vi "CloseCamera.vi"(8 "error in (no error)":errorcluster, 11 "HamaCam in":refnum<class "HamaCam.lvclass">) -> (0 "error out":errorcluster, 3 "HamaCam out":refnum<class "HamaCam.lvclass">)   [LabVIEW 2023, in "HamaCam.lvlib" / "HamaCam.lvclass"]
uses:
  HamaCam.lvclass
  HamaCam.lvclass/HamaCam.ctl
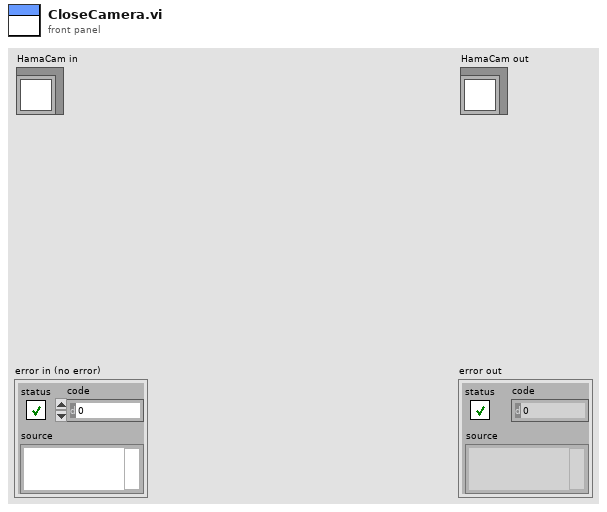
[diagram p1: front panel]
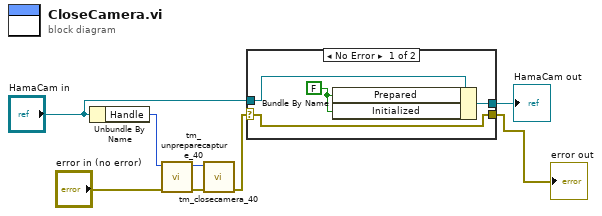
[diagram p0: block diagram]
diagram:
  n1 = Unbundle By Name("HamaCam in") -> ("Handle"=w6:u32)
  n2 = call "tm_unpreparecapture_40.vi"("error in (no error)"="error in (no error)", "Handle in"=w6) -> ("error out"=w8:errorcluster, "Handle out"=w7:u32)  [unwired: 8 in]
  n3 = call "tm_closecamera_40.vi"("error in (no error)"=w8, "Handle in"=w7) -> ("error out"=w4:errorcluster)  [unwired: 9 in]
  n4 = case shown="No Error" w4 {
    selector: w4 -> [w9 w13]
    tunnel: "HamaCam in" -> [w12 w14]
    tunnel: [w11 w14] -> w2
    tunnel: [w9 w13] -> w1
    frame No Error {
      w10 = FALSE ("CurrentState.Initialized")
      n5 = Bundle By Name(cluster=w12, "Prepared"=w10, "Initialized"=w10) -> (w11:refnum<class "HamaCam.lvclass">)
    }
    frame Error {
    }
  }
  "HamaCam out" <- w2
  "error out" <- w1
